vi "DS Activate PVProxy.vi"() -> ()   [LabVIEW 2016, in "CS++Utilities.lvlib"]
doc: "Activate or deactivate CS++PVProxy when using DataSocket."
uses:
  CS++Utilities.lvlib
panel:
  in  "Proxy-Activate URL":string="dstp://localhost/CSPP_Core_SV/myBaseProxy_Activate"
  in  "Activate?":bool=TRUE
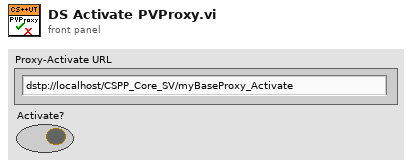
[diagram p1: front panel]
types:
  T1 = enum16{"Read", "Write", "ReadWrite", "BufferedRead", "BufferedReadWrite"}
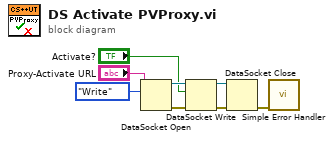
[diagram p0: block diagram]
diagram:
  n1 = DataSocket Open(10:T1."Write" ("mode"), 11:"Proxy-Activate URL") -> (0:w7:errorcluster, 3:w5:refnum<k13>)  [unwired: 2 in]
  n2 = DataSocket Write(8:w7, 10:"Activate?", 11:w5) -> (0:w3:errorcluster, 3:w2:refnum<k13>)  [unwired: 1 in, 1 out]
  n3 = DataSocket Close(8:w3, 11:w2) -> (0:w1:errorcluster)  [unwired: 1 in, 1 out]
  n4 = call <vilib>:"Simple Error Handler.vi"("error in (no error)"=w1) -> ()  [unwired: 4 in, 5 out]
